vi "Read Controller Details.vi"(8 "error in (no error)":errorcluster, 9 "Plugin File Path":path, 10 "Plugin Details in":T2, 11 "Refnum in":T1) -> (0 "error out":errorcluster, 2 "Plugin Details out 2":T2, 3 "refnum out":T1)   [LabVIEW 2020, in "Plugin Manager.lvlib"]
uses:
  Plugin Manager.lvlib
  Plugin Details.ctl
  Plugin Servers/Controller/Controller Type.ctl
  Plugin Types.ctl
  <vilib>/Utility/config.llb/Config Data RefNum.ctl
  <vilib>/Utility/config.llb/Read Key (String).vi
  <vilib>/Utility/config.llb/Read Key (Path).vi
  <vilib>/Utility/config.llb/NI_LVConfig.lvlib
  Plugin Servers/Controller/Generic Plugin.lvclass
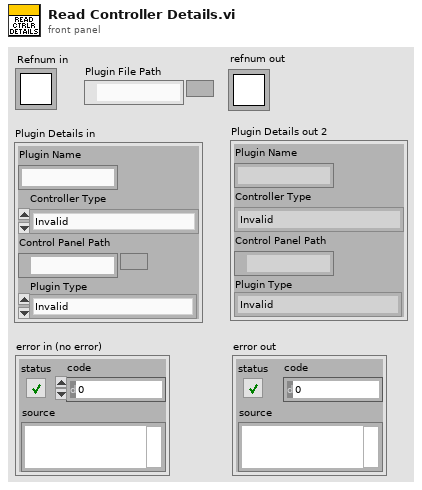
[diagram p1: front panel]
types:
  T1 = typedef "NI_LVConfig.lvlib/Config Data RefNum.ctl" = refnum<k1>
  T2 = typedef "Plugin Manager.lvlib/Plugin Details.ctl" = cluster{"Plugin Name":string, "Controller Type":T3, "Control Panel Path":path, "Plugin Type":T4}
  T3 = typedef "Generic Plugin.lvclass/Controller Type.ctl" = enum16{"Invalid", "Temperature Controller", "Pump Controller", "Generic Optimizer", "LC Parser"}
  T4 = typedef "Plugin Manager.lvlib/Plugin Types.ctl" = enum16{"Invalid", "Optimizer", "Analyzer", "Hardware"}
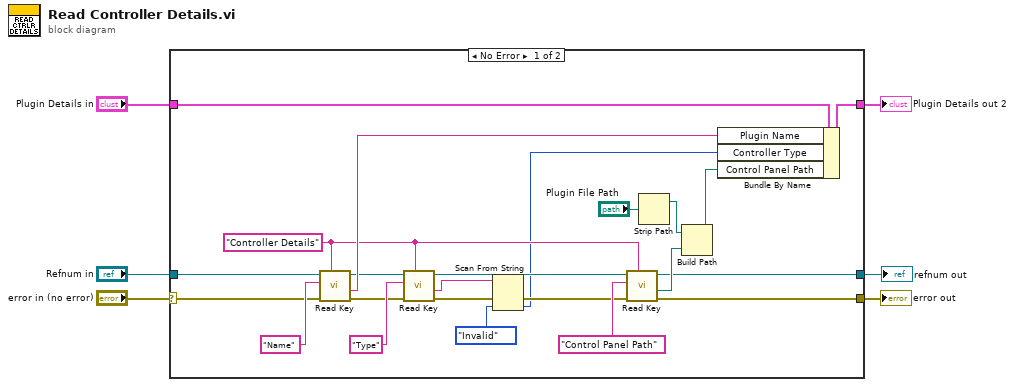
[diagram p0: block diagram]
diagram:
  n1 = case shown="No Error" "error in (no error)" {
    selector: "error in (no error)" -> [w14 w32]
    tunnel: "Plugin Details in" -> [w29 w30]
    tunnel: [w28 w30] -> w5
    tunnel: "Refnum in" -> [w26 w31]
    tunnel: [w7 w32] -> w3
    tunnel: [w16 w31] -> w2
    frame No Error {
      w21 = "Controller Details" ("section")
      n2 = call-poly <vilib>:"Read Key.vi"("section"=w21, "error in (no error)"=w14, "key"="Name", "refnum"=w26) -> ("error out"=w17:errorcluster, "value"=w27:string, "refnum out"=w18:T1)  [unwired: 4 in, 1 out]
      n3 = call-poly <vilib>:"Read Key.vi"("section"=w21, "error in (no error)"=w17, "key"="Type", "refnum"=w18) -> ("error out"=w12:errorcluster, "value"=w10:string, "refnum out"=w19:T1)  [unwired: 4 in, 1 out]
      n4 = Scan From String(input string=w10, error in=w12, default 1=Controller_Type."Invalid" ("Controller Type")) -> (error out=w11:errorcluster, output 1=w9:T3)  [unwired: 2 in, 2 out]
      n5 = call-poly <vilib>:"Read Key.vi"("section"=w21, "error in (no error)"=w11, "key"="Control Panel Path", "refnum"=w19) -> ("error out"=w7:errorcluster, "value"=w25:path, "refnum out"=w16:T1)  [unwired: 4 in, 1 out]
      n6 = Strip Path(path="Plugin File Path") -> (stripped path=w24:path)  [unwired: 1 out]
      n7 = Build Path(base path=w24, name or relative path=w25) -> (appended path=w8:path)
      n8 = Bundle By Name(cluster=w29, "Plugin Name"=w27, "Controller Type"=w9, "Control Panel Path"=w8) -> (w28:T2)
    }
    frame Error {
    }
  }
  "Plugin Details out 2" <- w5
  "error out" <- w3
  "refnum out" <- w2
